vi "Set Aircraft RC.vi"(8 "Error In":errorcluster, 10 "Aircraft RC Data":T1, 11 "Aircraft ID":u8) -> (0 "Error Out":errorcluster)   [LabVIEW 2014]
uses:
  Controls/Aircraft RC Data.ctl
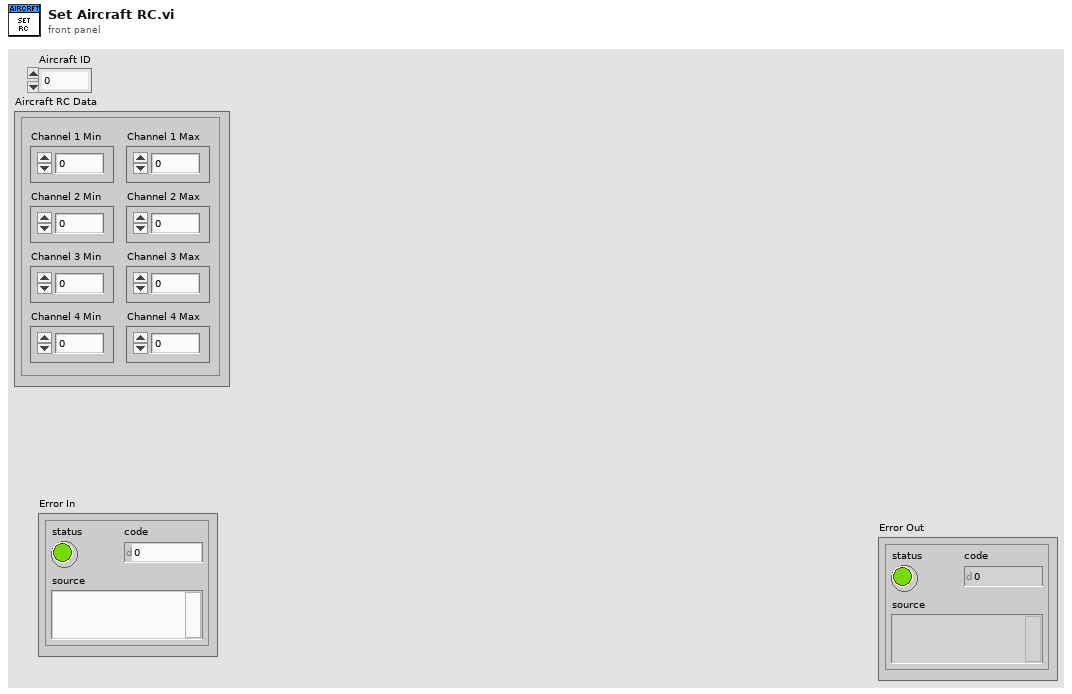
[diagram p1: front panel]
types:
  T1 = typedef "Aircraft RC Data.ctl" = cluster{"Channel 1 Min":i16, "Channel 1 Max":i16, "Channel 2 Min":i16, "Channel 2 Max":i16, "Channel 3 Min":i16, "Channel 3 Max":i16, "Channel 4 Min":i16, "Channel 4 Max":i16}
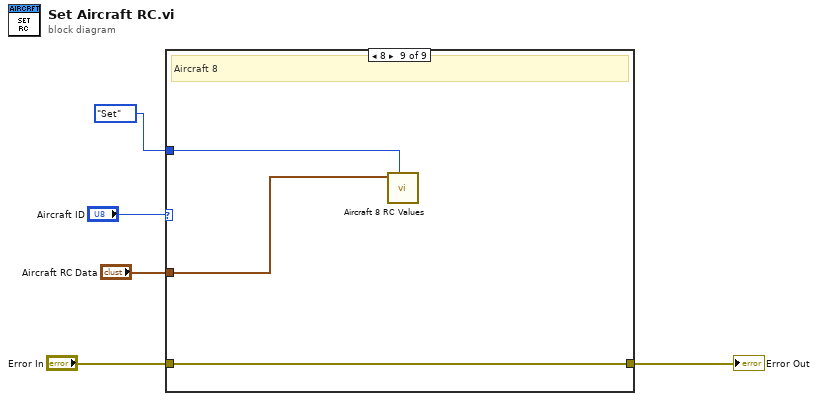
[diagram p0: block diagram]
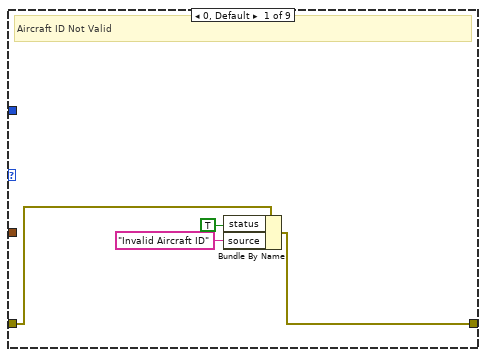
[diagram p2: hidden frame]
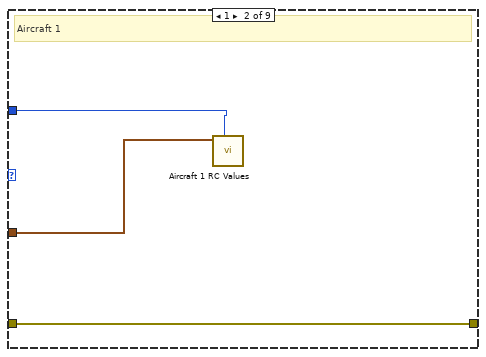
[diagram p3: hidden frame]
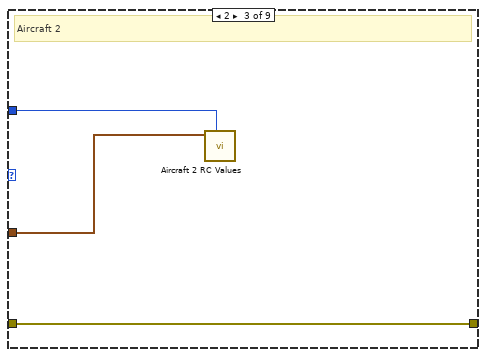
[diagram p4: hidden frame]
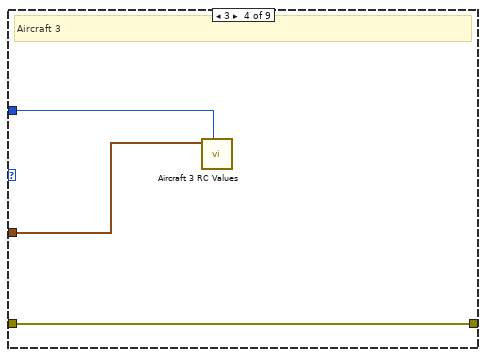
[diagram p5: hidden frame]
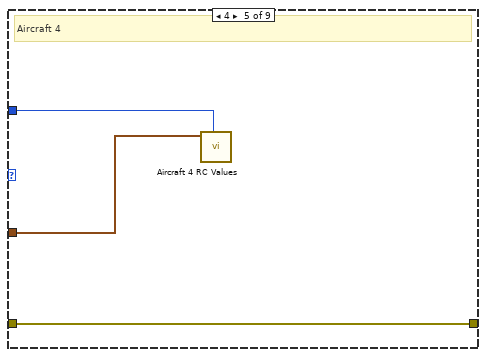
[diagram p6: hidden frame]
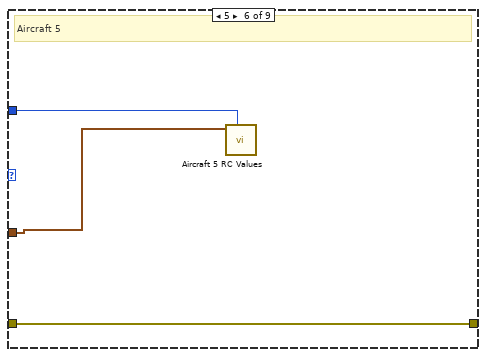
[diagram p7: hidden frame]
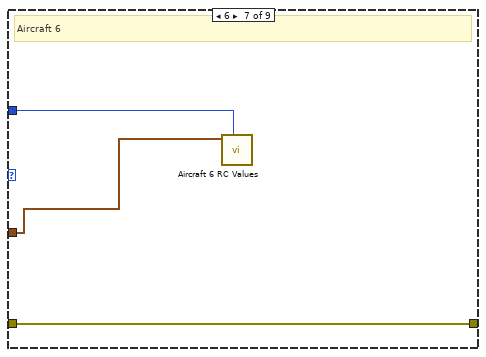
[diagram p8: hidden frame]
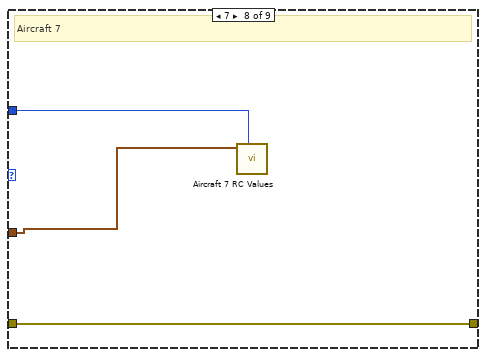
[diagram p9: hidden frame]
diagram:
  n1 = case shown="8" "Aircraft ID" {
    tunnel: [w8 w12 w15 w18 w21 w24 w27 w30 w33] -> w4
    tunnel: "Error In" -> [w9 w12 w15 w18 w21 w24 w27 w30 w33]
    tunnel: enum16{"Get", "Set"}."Set" ("Method") -> [_ w11 w14 w17 w20 w23 w26 w29 w32]
    tunnel: "Aircraft RC Data" -> [_ w10 w13 w16 w19 w22 w25 w28 w31]
    frame 0, Default {
      # "Aircraft ID Not Valid"
      n2 = Bundle By Name(cluster=w9, "status"=TRUE, "source"="Invalid Aircraft ID") -> (w8:errorcluster)
    }
    frame 1 {
      # "Aircraft 1"
      n3 = call "Aircraft 1 RC Values .vi"("Method"=w11, "Aircraft RC Data"=w10) -> ()  [unwired: 9 in, 1 out]
    }
    frame 2 {
      # "Aircraft 2"
      n4 = call "Aircraft 2 RC Values .vi"("Method"=w14, "Aircraft RC Data"=w13) -> ()  [unwired: 9 in, 1 out]
    }
    frame 3 {
      # "Aircraft 3"
      n5 = call "Aircraft 3 RC Values .vi"("Method"=w17, "Aircraft RC Data"=w16) -> ()  [unwired: 9 in, 1 out]
    }
    frame 4 {
      # "Aircraft 4"
      n6 = call "Aircraft 4 RC Values .vi"("Method"=w20, "Aircraft RC Data"=w19) -> ()  [unwired: 9 in, 1 out]
    }
    frame 5 {
      # "Aircraft 5"
      n7 = call "Aircraft 5 RC Values .vi"("Method"=w23, "Aircraft RC Data"=w22) -> ()  [unwired: 9 in, 1 out]
    }
    frame 6 {
      # "Aircraft 6"
      n8 = call "Aircraft 6 RC Values .vi"("Method"=w26, "Aircraft RC Data"=w25) -> ()  [unwired: 9 in, 1 out]
    }
    frame 7 {
      # "Aircraft 7"
      n9 = call "Aircraft 7 RC Values .vi"("Method"=w29, "Aircraft RC Data"=w28) -> ()  [unwired: 9 in, 1 out]
    }
    frame 8 {
      # "Aircraft 8"
      n10 = call "Aircraft 8 RC Values .vi"("Method"=w32, "Aircraft RC Data"=w31) -> ()  [unwired: 9 in, 1 out]
    }
  }
  "Error Out" <- w4
